vi "SVFA Unit Conversion (XY) (1 Ch).vi"(0 "magnitudes":cluster{"time/rev/rpm":dbl[], "magnitude":dbl[]} {"magnitude" format="%.2f"; "time/rev/rpm" format="%.2f"}, 1 "desired scaling":T1 {"dB reference (0: no change)" format="%.2f"}, 4 "magnitude info in":T2={"channel name"="", "description"="", "x-axis units"=0, "spectral info"={"spectrum type"=enum."Power [Magnitude^2]", "linear/dB"=enum."linear", "window"=0, "window size"=0, "FFT size"=0}, "engineering units"=0, "custom label"="", "dB reference [EU]"=0.0, "peak units"=enum."rms", "weighting filter"=0, "spectral density?"=FALSE, "unit label"="", "spectrum skewed?"=FALSE, "complimentary spectrum units"=enum."none"} {"x-axis units" items=["Time (s)"=0, "Frequency-CB (Hz)"=1, "Frequency-CPB (Hz)"=1248, "Frequency-Arbitrary (Hz)"=2357, "Quefrency (s)"=2, "Revolutions (rev)"=3, "Order"=4, "Speed (RPM)"=11, "Speed (rad/s)"=21, "Index"=65535]; "weighting filter" items=["Linear", "A-weighting", "B-weighting", "C-weighting", "ITU-R 468-4", "Dolby", "CCITT", "C-message", "Wb", "Wc", "Wd", "We", "Wf", "Wh", "Wj", "Wk", "Wm", "AES17 20 kHz lowpass", "AES17 40 kHz lowpass", "AES17 20 kHz highpass", "AES17 40 kHz highpass"]; "dB reference [EU]" format="%.2f"; "engineering units" items=["custom..."=0, "V"=1, "A"=21, "C"=30, "pC"=31, "s"=32, "-"=29, "Pa"=2, "N"=20, "g"=3, "m/s^2"=4, "m/s"=5, "m"=6, "mm/s"=12, "mm"=13, "micron/s"=14, "micron"=15, "in/s^2"=7, "in/s"=8, "in"=9, "mil/s"=10, "mil"=11, "rad/s^2"=16, "rad/s"=17, "rad"=18, "deg/s^2"=26, "deg/s"=27, "deg"=28, "RPM"=22, "cycle/s^2"=23, "Hz"=24, "cycle"=25, "strain"=19]; "spectral info"."window" items=["None "=0, "Hanning"=1, "Hamming"=2, "Blackman-Harris"=3, "Exact Blackman"=4, "Blackman"=5, "Flat Top"=6, "4 Term B-Harris "=7, "7 Term B-Harris"=8, "Low Sidelobe"=9, "Force - Exponential"=10, "Gaussian"=62]}, 5 "error in (no error)":errorcluster) -> (14 "converted magnitudes":cluster{"time/rev/rpm":dbl[], "magnitude":dbl[]} {"magnitude" format="%.2f"; "time/rev/rpm" format="%.2f"}, 15 "unit label":string, 18 "magnitude info out":T2={"channel name"="", "description"="", "x-axis units"=0, "spectral info"={"spectrum type"=enum."Power [Magnitude^2]", "linear/dB"=enum."linear", "window"=0, "window size"=0, "FFT size"=0}, "engineering units"=0, "custom label"="", "dB reference [EU]"=0.0, "peak units"=enum."rms", "weighting filter"=0, "spectral density?"=FALSE, "unit label"="", "spectrum skewed?"=FALSE, "complimentary spectrum units"=enum."none"} {"x-axis units" items=["Time (s)"=0, "Frequency-CB (Hz)"=1, "Frequency-CPB (Hz)"=1248, "Frequency-Arbitrary (Hz)"=2357, "Quefrency (s)"=2, "Revolutions (rev)"=3, "Order"=4, "Speed (RPM)"=11, "Speed (rad/s)"=21, "Index"=65535]; "weighting filter" items=["Linear", "A-weighting", "B-weighting", "C-weighting", "ITU-R 468-4", "Dolby", "CCITT", "C-message", "Wb", "Wc", "Wd", "We", "Wf", "Wh", "Wj", "Wk", "Wm", "AES17 20 kHz lowpass", "AES17 40 kHz lowpass", "AES17 20 kHz highpass", "AES17 40 kHz highpass"]; "dB reference [EU]" format="%.2f"; "engineering units" items=["custom..."=0, "V"=1, "A"=21, "C"=30, "pC"=31, "s"=32, "-"=29, "Pa"=2, "N"=20, "g"=3, "m/s^2"=4, "m/s"=5, "m"=6, "mm/s"=12, "mm"=13, "micron/s"=14, "micron"=15, "in/s^2"=7, "in/s"=8, "in"=9, "mil/s"=10, "mil"=11, "rad/s^2"=16, "rad/s"=17, "rad"=18, "deg/s^2"=26, "deg/s"=27, "deg"=28, "RPM"=22, "cycle/s^2"=23, "Hz"=24, "cycle"=25, "strain"=19]; "spectral info"."window" items=["None "=0, "Hanning"=1, "Hamming"=2, "Blackman-Harris"=3, "Exact Blackman"=4, "Blackman"=5, "Flat Top"=6, "4 Term B-Harris "=7, "7 Term B-Harris"=8, "Low Sidelobe"=9, "Force - Exponential"=10, "Gaussian"=62]}, 19 "error out":errorcluster)   [LabVIEW 2017]
doc: "Converts between dB/linear, magnitude/magnitude^2, rms/peak/peak-peak, spectrum/spectral density, and dB ref1/dB ref2. Wire data to the <B>spectrum</B> input to determine the polymorphic instance to use or manually select the instance."
uses:
  <vilib>/addons/_NISVFA/_Shared subVIs/Controls/svc_Spectrum Info.ctl
  <vilib>/addons/_NISVFA/_Shared subVIs/Controls/svc_X-Axis Units.ctl
  <vilib>/addons/_NISVFA/_Shared subVIs/Controls/svc_Spectrum Type.ctl
  <vilib>/addons/_NISVFA/_Shared subVIs/Controls/svc_Engineering Units Text Ring.ctl
  <vilib>/addons/_NISVFA/_Shared subVIs/Controls/svc_Weighting Filter Text Ring.ctl
  <vilib>/addons/_NISVFA/_Shared subVIs/Controls/svc_Complimentary Spectrum Units.ctl
  <vilib>/addons/_NISVFA/_Spectrum Processing/subVIs/svfa_Peak to RMS to Peak2Peak.vi
  <vilib>/addons/_NISVFA/_Spectrum Processing/subVIs/svfa_Mag to Mag2.vi
  <vilib>/addons/_NISVFA/_Spectrum Processing/subVIs/svfa_Linear to dB.vi
  <vilib>/addons/_NISVFA/_Spectrum Processing/subVIs/svfa_dBrefA to dBrefB.vi
  <vilib>/addons/_NISVFA/_Spectrum Processing/subVIs/svfa_Spectrum to Spectral Density.vi
  <vilib>/addons/_NISVFA/_Shared subVIs/Common/svc_Get Weighting Enum and Labels.vi
  <vilib>/addons/_NISVFA/_Shared subVIs/Common/svc_Unit Label Lexical Class.vi
  <vilib>/addons/_NISVFA/_Shared subVIs/Common/svc_Engineering Units to Unit Label.vi
  <vilib>/addons/_NISVFA/_Shared subVIs/Common/svc_Format Value (DBL).vi
  <vilib>/addons/_NISVFA/_Shared subVIs/Common/svc_Window Parameters.vi
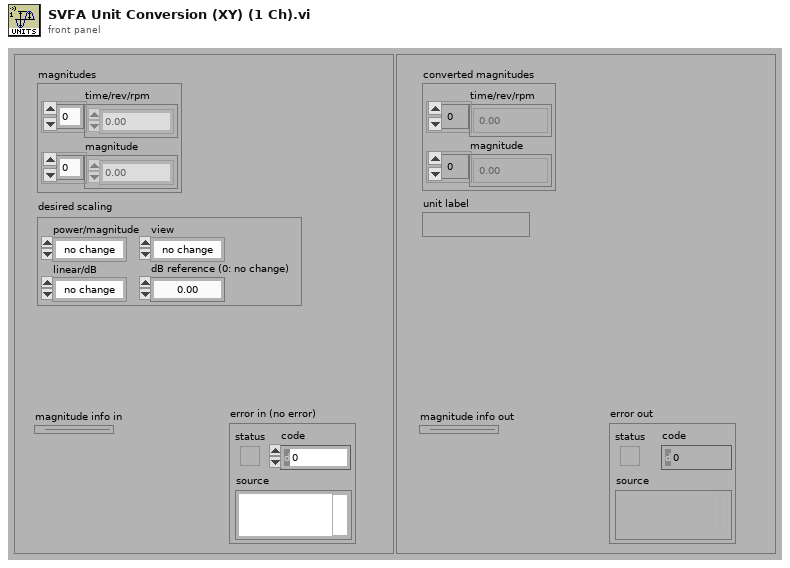
[diagram p1: front panel]
types:
  T1 = cluster{"linear/dB":enum16{"no change", "linear", "dB"}, "dB reference (0: no change)":dbl, "power/magnitude":enum16{"no change", "power", "magnitude"}, "view":enum16{"no change", "rms", "peak", "peak-peak"}}
  T2 = typedef "svc_Spectrum Info.ctl" = cluster{"channel name":string, "description":string, "x-axis units":T3, "spectral info":cluster{"spectrum type":T4, "linear/dB":enum16{"linear", "dB"}, "window":u16, "window size":i32, "FFT size":i32}, "engineering units":T5, "custom label":string, "dB reference [EU]":dbl, "peak units":enum16{"rms", "peak", "peak-peak"}, "weighting filter":T6, "spectral density?":bool, "unit label":string, "spectrum skewed?":bool, "complimentary spectrum units":T7}
  T3 = typedef "svc_X-Axis Units.ctl" = u16
  T4 = typedef "svc_Spectrum Type.ctl" = enum16{"FFT Spectrum [complex]", "Amplitude [Magnitude]", "Power [Magnitude^2]", "Cross Spectrum [complex]", "Frequency Response [Complex]"}
  T5 = typedef "svc_Engineering Units Text Ring.ctl" = u16
  T6 = typedef "svc_Weighting Filter Text Ring.ctl" = u16
  T7 = typedef "svc_Complimentary Spectrum Units.ctl" = enum16{"none", "radians", "degrees", "cycles", "imaginary"}
  T8 = enum16{"no change", "spectrum", "spectral density"}
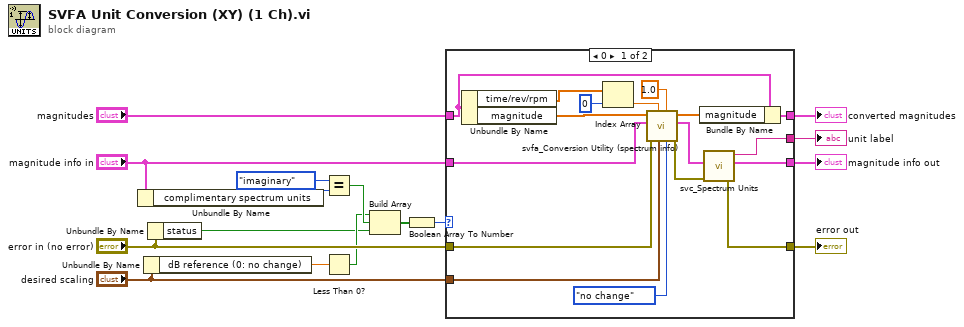
[diagram p0: block diagram]
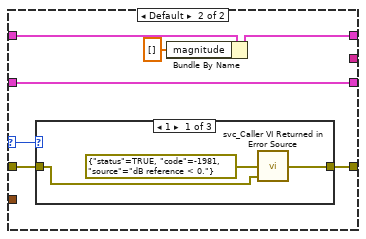
[diagram p2: hidden frame]
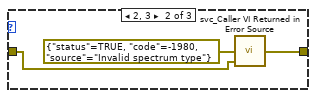
[diagram p3: hidden frame]
diagram:
  n1 = Unbundle By Name("magnitude info in") -> ("complimentary spectrum units"=w5:T7)
  n2 = Unbundle By Name("desired scaling") -> ("dB reference (0: no change)"=w9:dbl)
  n3 = Unbundle By Name("error in (no error)") -> ("status"=w3:bool)
  n4 = Equal?(x=svc_Complimentary_Spectrum_Units."imaginary" ("y"), y=w5) -> (x = y?=w8:bool)
  n5 = Less Than 0?(x=w9) -> (x < 0?=w7:bool)
  n6 = Build Array(w7, w8, w3) -> (w4:bool[])
  n7 = Boolean Array To Number(Boolean array=w4) -> (number=w2:u32)
  n8 = case shown="0" w2 {
    selector: w2 -> [_ w40]
    tunnel: "magnitudes" -> [w33 w36]
    tunnel: [w32 w35] -> w14
    tunnel: [w31 w38] -> w1
    tunnel: [w30 _] -> w10
    tunnel: [w29 w37] -> w11
    tunnel: "magnitude info in" -> [w28 w37]
    tunnel: "desired scaling" -> [w27 _]
    tunnel: "error in (no error)" -> [w19 w39]
    frame 0 {
      n9 = Unbundle By Name(w33) -> ("time/rev/rpm"=w23:dbl[], "magnitude"=w25:dbl[])
      n10 = Index Array(array=w23, index=0) -> (element=w21:dbl)
      n11 = call <vilib>:"svfa_Conversion Utility (spectrum info).vi"("spectral density desired"=T8."no change", "dx"=1.0 ("index"), "desired scaling"=w27, "x0"=w21, "error in (no error)"=w19, "spectrum info in"=w28, "input signal"=w25) -> ("error out"=w17:errorcluster, "spectrum info out"=w24:T2, "converted signal"=w26:dbl[])  [unwired: 2 in]
      n12 = Bundle By Name(cluster=w33, "magnitude"=w26) -> (w32:cluster{"time/rev/rpm":dbl[], "magnitude":dbl[]})
      n13 = call <vilib>:"svc_Spectrum Units.vi"("error in (no error)"=w17, "spectrum info in"=w24) -> ("error out"=w31:errorcluster, "spectrum info out"=w29:T2, "unit label"=w30:string)  [unwired: 2 in, 1 out]
    }
    frame Default {
      n14 = case shown="1" w40 {
        tunnel: w39 -> [w42 w44 w47]
        tunnel: [w41 w46 w47] -> w38
        frame 1 {
          n15 = call <vilib>:"svc_Caller VI Returned in Error Source.vi"("warning input to caller"=w42, "error in (no error)"=errorcluster {"status"=TRUE, "code"=-1981, "source"="dB reference < 0."} ("error out")) -> ("error out"=w41:errorcluster)  [unwired: 3 in]
        }
        frame 2, 3 {
          n16 = call <vilib>:"svc_Caller VI Returned in Error Source.vi"("warning input to caller"=w44, "error in (no error)"=errorcluster {"status"=TRUE, "code"=-1980, "source"="Invalid spectrum type"} ("error out")) -> ("error out"=w46:errorcluster)  [unwired: 3 in]
        }
        frame 4.., Default {
        }
      }
      n17 = Bundle By Name(cluster=w36, "magnitude"=dbl[] []) -> (w35:cluster{"time/rev/rpm":dbl[], "magnitude":dbl[]})
    }
  }
  "error out" <- w1
  "converted magnitudes" <- w14
  "magnitude info out" <- w11
  "unit label" <- w10
